vi "PathfinderUtil_OptimizeTrajectoryStates.vi"(11 "inputTrajectoryStates":T1[](array[typedef]) {"POSE"."ROTATION"."SIN" format="%13.4f"; "POSE"."ROTATION"."COS" format="%13.4f"; "POSE"."ROTATION"."VALUE" format="%13.4f"; "POSE"."TRANSLATION"."Y" format="%14.3f"; "POSE"."TRANSLATION"."X" format="%14.3f"}) -> (3 "outputTrajectoryStates":T1[](array[typedef]) {"POSE"."ROTATION"."SIN" format="%13.4f"; "POSE"."ROTATION"."COS" format="%13.4f"; "POSE"."ROTATION"."VALUE" format="%13.4f"; "POSE"."TRANSLATION"."Y" format="%14.3f"; "POSE"."TRANSLATION"."X" format="%14.3f"})   [LabVIEW 2019, in "Trajectory_Library.lvlib"]
doc: "Optimize trajectory states by removing states that are too similar. The first and last states are always kept. This reduces the overall number of states. This also prevents potential divide by zero errors during sample interpoloation. This is used when convering a Pathfinder Path to a Trajectory."
uses:
  Trajectory_Library.lvlib
  TypeDef/TRANSLATION2D.ctl
  TypeDef/ROTATION2D.ctl
  TypeDef/POSE2D.ctl
  TypeDef/TRAJ_STATE.ctl
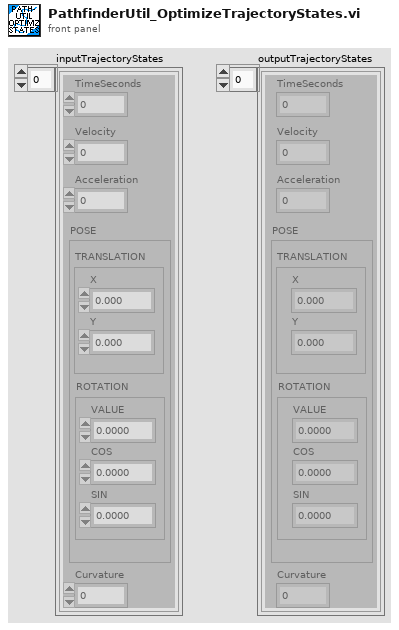
[diagram p1: front panel]
types:
  T1 = typedef "Trajectory_Library.lvlib/TRAJ_STATE.ctl" = cluster{"TimeSeconds":dbl, "Velocity":dbl, "Acceleration":dbl, "POSE":T2, "Curvature":dbl}
  T2 = typedef "Trajectory_Library.lvlib/POSE2D.ctl" = cluster{"TRANSLATION":T3, "ROTATION":T4}
  T3 = typedef "Trajectory_Library.lvlib/TRANSLATION2D.ctl" = cluster{"X":dbl, "Y":dbl}
  T4 = typedef "Trajectory_Library.lvlib/ROTATION2D.ctl" = cluster{"VALUE":dbl, "COS":dbl, "SIN":dbl}
  T5 = typedef "WPILib_Math.lvlib/TWIST2D.ctl" = cluster{"dX":dbl, "dY":dbl, "dTHETA":dbl}
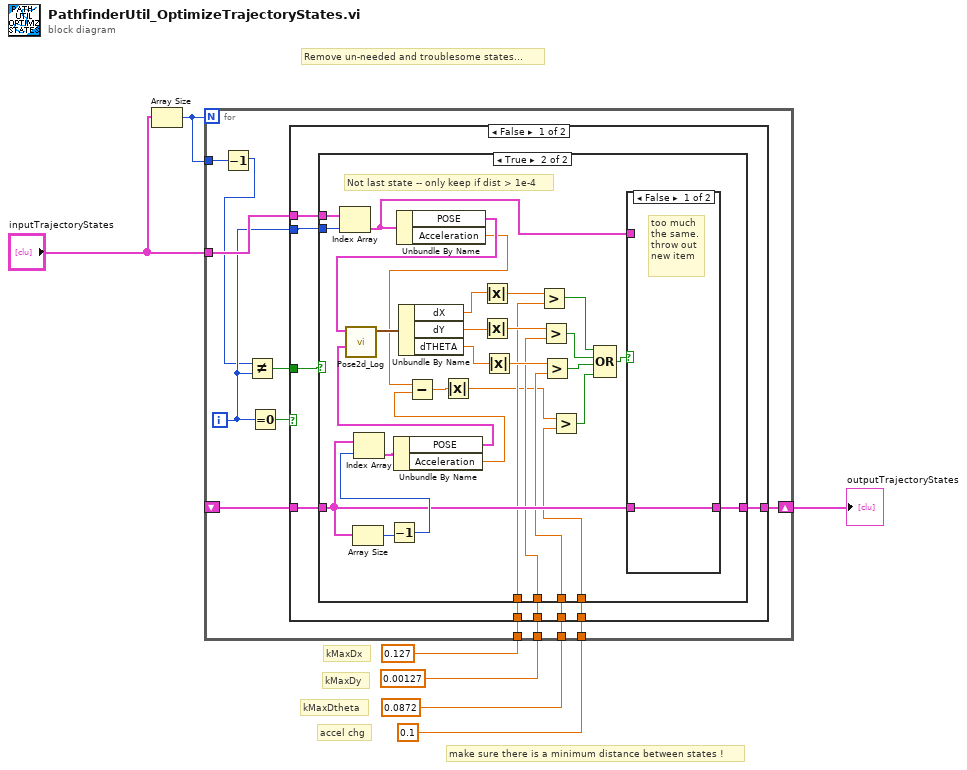
[diagram p0: block diagram]
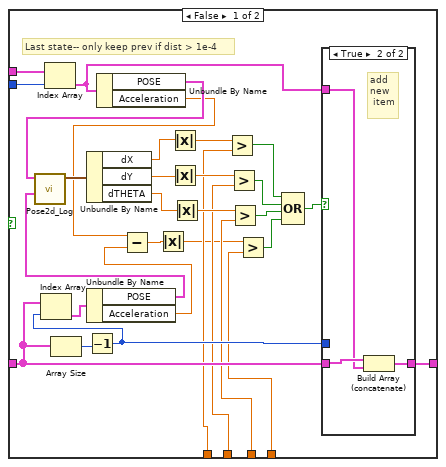
[diagram p2: hidden frame]
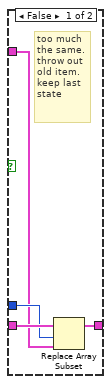
[diagram p3: hidden frame]
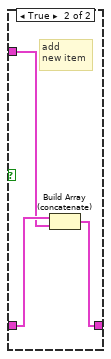
[diagram p4: hidden frame]
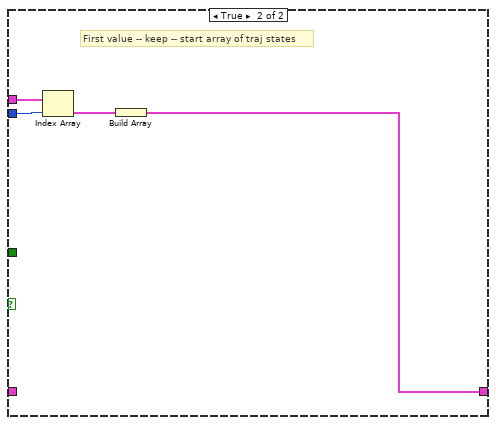
[diagram p5: hidden frame]
diagram:
  # "Remove un-needed and troublesome states..."
  # "accel chg"
  # "kMaxDtheta"
  # "kMaxDy"
  # "kMaxDx"
  # "make sure there is a minimum distance between states !"
  n1 = Array Size(array="inputTrajectoryStates") -> (size(s)=w3:i32)
  n2 = for {
    N: w3 -> [_]
    tunnel: "inputTrajectoryStates" -> [w18]
    shift-right: [w17] -> w2
    shift-left: _ -> [w16]
    tunnel: w3 -> [w15]
    tunnel: 0.127 -> [w11]
    tunnel: 0.00127 -> [w10]
    tunnel: 0.0872 -> [w9]
    tunnel: 0.1 -> [w8]
    i -> [w14]
    n3 = Decrement(x=w15) -> (x-1=w13:i32)
    n4 = Not Equal?(x=w13, y=w14) -> (x != y?=w12:bool)
    n5 = Equal To 0?(x=w14) -> (x = 0?=w19:bool)
    n6 = case shown="False" w19 {
      tunnel: w18 -> [w27 w103]
      tunnel: w14 -> [w26 w102]
      tunnel: [w24 w100] -> w17
      tunnel: w16 -> [w25 _]
      tunnel: w12 -> [w28 _]
      tunnel: w11 -> [w23 _]
      tunnel: w10 -> [w22 _]
      tunnel: w9 -> [w21 _]
      tunnel: w8 -> [w20 _]
      frame False {
        n7 = case shown="True" w28 {
          tunnel: w27 -> [w57 w95]
          tunnel: w26 -> [w56 w94]
          tunnel: w25 -> [w55 w91]
          tunnel: [w54 w90] -> w24
          tunnel: w23 -> [w37 w74]
          tunnel: w22 -> [w36 w73]
          tunnel: w21 -> [w35 w72]
          tunnel: w20 -> [w29 w70]
          frame False {
            # "Last state-- only keep prev if dist > 1e-4"
            n8 = Index Array(array=w57, index=w56) -> (element=w39:T1)
            n9 = Array Size(array=w55) -> (size(s)=w58:i32)
            n10 = Decrement(x=w58) -> (x-1=w53:i32)
            n11 = Index Array(array=w55, index=w53) -> (element=w41:T1)
            n12 = Unbundle By Name(w41) -> ("POSE"=w40:T2, "Acceleration"=w30:dbl)
            n13 = Unbundle By Name(w39) -> ("POSE"=w38:T2, "Acceleration"=w31:dbl)
            n14 = call "Pose2d_Log.vi"("end POSE"=w40, "in POSE"=w38) -> ("out TWIST"=w52:T5)  [unwired: 9 in]
            n15 = Unbundle By Name(w52) -> ("dX"=w45:dbl, "dY"=w44:dbl, "dTHETA"=w43:dbl)
            n16 = Subtract(x=w31, y=w30) -> (x-y=w34:dbl)
            n17 = Absolute Value(x=w34) -> (abs(x)=w32:dbl)
            n18 = Absolute Value(x=w45) -> (abs(x)=w51:dbl)
            n19 = Absolute Value(x=w44) -> (abs(x)=w50:dbl)
            n20 = Absolute Value(x=w43) -> (abs(x)=w49:dbl)
            n21 = Greater?(x=w51, y=w37) -> (0:w46:bool)
            n22 = Greater?(x=w50, y=w36) -> (0:w47:bool)
            n23 = Greater?(x=w49, y=w35) -> (0:w48:bool)
            n24 = Greater?(x=w32, y=w29) -> (0:w33:bool)
            n25 = Compound Arithmetic op=OR(w46, w47, w48, w33) -> (w42:bool)
            n26 = case shown="True" w42 {
              tunnel: w55 -> [w62 w64]
              tunnel: w39 -> [w60 w63]
              tunnel: [w59 w65] -> w54
              tunnel: w53 -> [w61 _]
              frame False {
                # "too much\nthe same.\nthrow out\nold item.\nkeep last \nstate"
                n27 = Replace Array Subset(array=w62, new element=w60, index=w61) -> (w59:T1[])
              }
              frame True {
                # "add\nnew\n item"
                n28 = Build Array (concatenate)(w64, w63) -> (w65:T1[])
              }
            }
          }
          frame True {
            # "Not last state -- only keep if dist > 1e-4"
            n29 = Index Array(array=w95, index=w94) -> (element=w88:T1)
            n30 = Array Size(array=w91) -> (size(s)=w93:i32)
            n31 = Decrement(x=w93) -> (x-1=w92:i32)
            n32 = Index Array(array=w91, index=w92) -> (element=w89:T1)
            n33 = Unbundle By Name(w89) -> ("POSE"=w86:T2, "Acceleration"=w67:dbl)
            n34 = Unbundle By Name(w88) -> ("POSE"=w87:T2, "Acceleration"=w66:dbl)
            n35 = call "Pose2d_Log.vi"("end POSE"=w86, "in POSE"=w87) -> ("out TWIST"=w85:T5)  [unwired: 9 in]
            n36 = Unbundle By Name(w85) -> ("dX"=w77:dbl, "dY"=w76:dbl, "dTHETA"=w75:dbl)
            n37 = Subtract(x=w66, y=w67) -> (x-y=w69:dbl)
            n38 = Absolute Value(x=w69) -> (abs(x)=w68:dbl)
            n39 = Absolute Value(x=w77) -> (abs(x)=w84:dbl)
            n40 = Absolute Value(x=w76) -> (abs(x)=w83:dbl)
            n41 = Absolute Value(x=w75) -> (abs(x)=w82:dbl)
            n42 = Greater?(x=w84, y=w74) -> (0:w79:bool)
            n43 = Greater?(x=w83, y=w73) -> (0:w80:bool)
            n44 = Greater?(x=w82, y=w72) -> (0:w81:bool)
            n45 = Greater?(x=w68, y=w70) -> (0:w71:bool)
            n46 = Compound Arithmetic op=OR(w79, w80, w81, w71) -> (w78:bool)
            n47 = case shown="False" w78 {
              tunnel: w91 -> [w96 w98]
              tunnel: w88 -> [_ w97]
              tunnel: [w96 w99] -> w90
              frame False {
                # "too much\nthe same.\nthrow out\nnew item"
              }
              frame True {
                # "add\nnew item"
                n48 = Build Array (concatenate)(w98, w97) -> (w99:T1[])
              }
            }
          }
        }
      }
      frame True {
        # "First value -- keep -- start array of traj states"
        n49 = Index Array(array=w103, index=w102) -> (element=w101:T1)
        n50 = Build Array(w101) -> (w100:T1[])
      }
    }
  }
  "outputTrajectoryStates" <- w2
